vi "cs_saveStimParam.vi"(0 "Total Trials":i32, 1 "Trial Randomization":enum32{"50% exactly", "Radio Selection 2"}(radio), 2 "Go Trial S#":i32=3, 3 "NoGo Trial S#":i32=4, 4 "Stims 1":dbl[][](array[numeric]), 5 "Stims 2":dbl[][](array[numeric]), 9 "error in (no error)":errorcluster) -> (10 "Path":path, 13 "error out":errorcluster)   [LabVIEW 2012]
uses:
  <vilib>/Utility/xml.llb/Write to XML File(array).vi
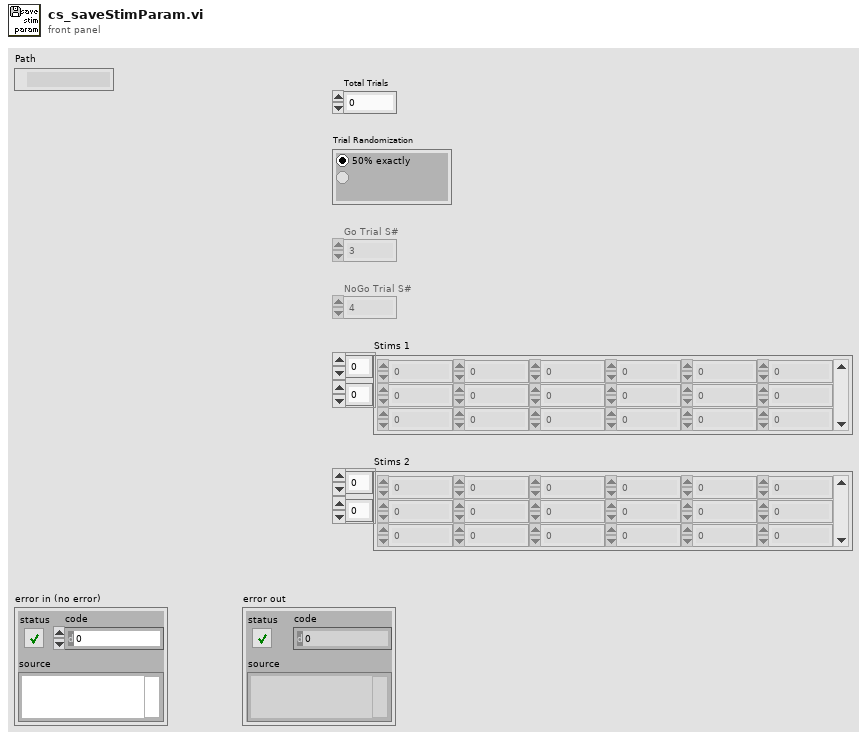
[diagram p1: front panel]
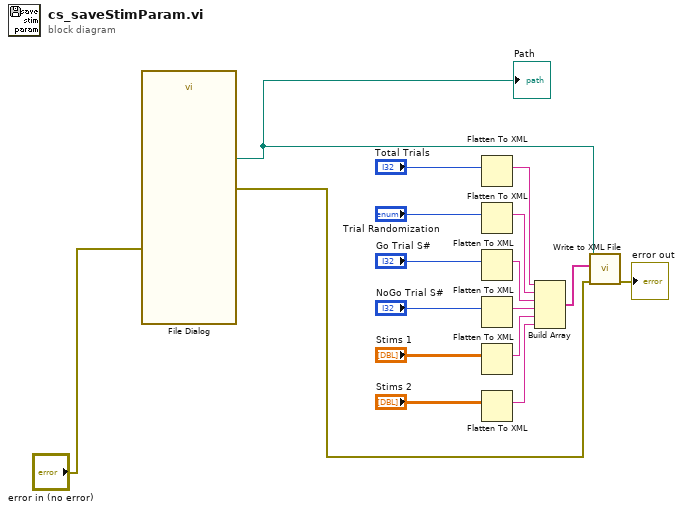
[diagram p0: block diagram]
diagram:
  n1 = call "File Dialog"("error in"="error in (no error)") -> ("selected path"=w16:path, "error out"=w14:errorcluster)  [unwired: 11 in, 2 out]
  "Path" <- w16
  n2 = Flatten To XML(anything="Total Trials") -> (xml string=w7:string)
  n3 = Flatten To XML(anything="Trial Randomization") -> (xml string=w6:string)
  n4 = Flatten To XML(anything="Go Trial S#") -> (xml string=w5:string)
  n5 = Flatten To XML(anything="NoGo Trial S#") -> (xml string=w4:string)
  n6 = Flatten To XML(anything="Stims 1") -> (xml string=w3:string)
  n7 = Flatten To XML(anything="Stims 2") -> (xml string=w2:string)
  n8 = Build Array(w7, w6, w5, w4, w3, w2) -> (w1:string[])
  n9 = call-poly <vilib>:"Write to XML File.vi"("error in (no error)"=w14, "XML Input"=w1, "XML File Path"=w16) -> ("error out"=→"error out":errorcluster)  [unwired: 6 in, 2 out]
